vi "Write Period in ms.vi"(8 "error in (no error)":errorcluster, 10 "Period in ms":u32, 11 "Poll Msg in":refnum<class "Poll Msg.lvclass">) -> (0 "error out":errorcluster, 3 "Poll Msg out":refnum<class "Poll Msg.lvclass">)   [LabVIEW 2024, in "Poll Msg.lvclass"]
uses:
  Poll Msg.lvclass
  Poll Msg.lvclass/Poll Msg.ctl
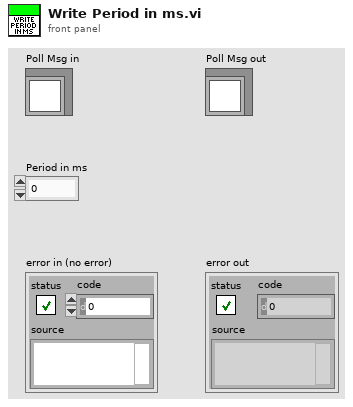
[diagram p1: front panel]
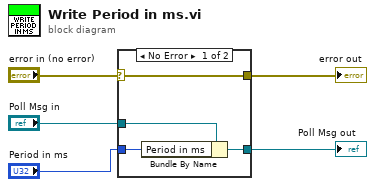
[diagram p0: block diagram]
diagram:
  n1 = case shown="No Error" "error in (no error)" {
    selector: "error in (no error)" -> [w9 w10]
    tunnel: [w9 w10] -> w4
    tunnel: [w7 w11] -> w2
    tunnel: "Poll Msg in" -> [w8 w11]
    tunnel: "Period in ms" -> [w6 _]
    frame No Error {
      n2 = Bundle By Name(cluster=w8, "Period in ms"=w6) -> (w7:refnum<class "Poll Msg.lvclass">)
    }
    frame Error {
    }
  }
  "error out" <- w4
  "Poll Msg out" <- w2
